vi "LFU Set File Pointer__ogtk.vi"(4 "error in (no error)":errorcluster, 5 "offset in (0)":dbl, 6 "pos mode (current)":enum16{"start", "end", "current"}(ring)=enum."current", 7 "handle":u32) -> (0 "error out":errorcluster, 1 "offset out":dbl, 3 "handle out":u32)   [LabVIEW 2018]
doc: "Low level utility function to change the current read/write pointer in a file using a double precision number to work for files larger than 2GB."
uses:
  kernel32.dll
panel:
  # "max offset is limited to about\n2^51 (1 000 000 000 000 000)  bytes\nto maintain full resolution of 1 bytes"
  # "LFU Set File Pointer.vi\n\nPlease visit http://www.OpenG.org to learn about the\nOpen Source LabVIEW software movement.\n\nNOTICE -- YOU MUST LEAVE THIS NOTICE IN PLACE.  PER THE TERMS OF THE LICENSE BELOW, YOU MAY SUBLICENSE THIS SOFTWARE \nIN ANY WAY THAT DOES NOT CONFLICT WITH THIS LICENSE.\n\n### BSD License (http://www.opensource.org/licenses/bsd-license.php) Begin ###\n\nCopyright (c) 2003, Rolf Kalbermatter <rolf.kalbermatter@citeng.com>\n\nAll rights reserved.\n\nRedistribution and use in source and binary forms, with or without modification, are permitted provided that the following conditions are met:\n\n    * Redistributions of source code must retain the above copyright notice, this list of conditions and the following disclaimer.\n    * Redistributions in binary form must reproduce the above copyright notice, this list of conditions and the following disclaimer in the \n       documentation and/or other materials provided with the distribution.\n    * Neither the name of SciWare, James Kring, Inc., nor the names of its contributors may be used to endorse or promote products derived \n       from this software without specific prior written permission.\n\nTHIS SOFTWARE IS PROVIDED BY THE COPYRIGHT HOLDERS AND CONTRIBUTORS \"AS IS\" AND ANY EXPRESS OR IMPLIED WARRANTIES, \nINCLUDING, BUT NOT LIMITED TO, THE IMPLIED WARRANTIES OF MERCHANTABILITY AND FITNESS FOR A PARTICULAR PURPOSE ARE \nDISCLAIMED. IN NO EVENT SHALL THE COPYRIGHT OWNER OR CONTRIBUTORS BE LIABLE FOR ANY DIRECT, INDIRECT, INCIDENTAL,\n SPECIAL, EXEMPLARY, OR CONSEQUENTIAL DAMAGES (INCLUDING, BUT NOT LIMITED TO, PROCUREMENT OF SUBSTITUTE GOODS OR \nSERVICES; LOSS OF USE, DATA, OR PROFITS; OR BUSINESS INTERRUPTION) HOWEVER CAUSED AND ON ANY THEORY OF LIABILITY, \nWHETHER IN CONTRACT, STRICT LIABILITY, OR TORT (INCLUDING NEGLIGENCE OR OTHERWISE) ARISING IN ANY WAY OUT OF THE USE \nOF THIS SOFTWARE, EVEN IF ADVISED OF THE POSSIBILITY OF SUCH DAMAGE.\n\n### BSD License End ###"
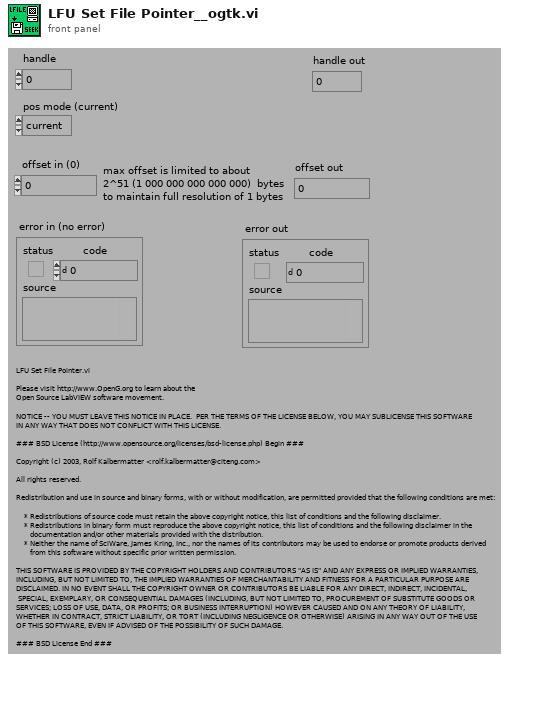
[diagram p1: front panel]
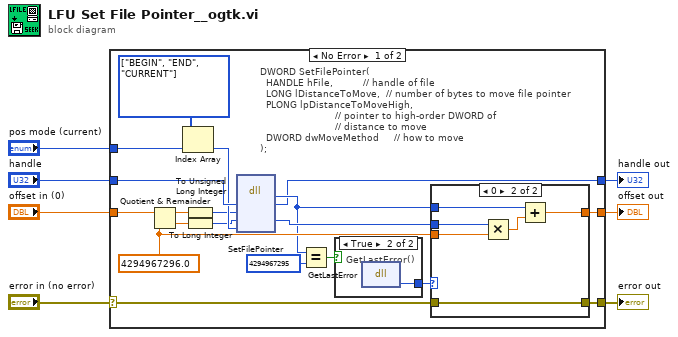
[diagram p0: block diagram]
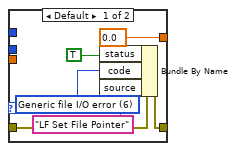
[diagram p2: hidden frame]
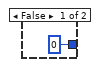
[diagram p3: hidden frame]
diagram:
  n1 = case shown="No Error" "error in (no error)" {
    selector: "error in (no error)" -> [w23 w41]
    tunnel: [w13 w43] -> w7
    tunnel: "handle" -> [w12 w43]
    tunnel: "pos mode (current)" -> [w26 _]
    tunnel: "offset in (0)" -> [w25 w42]
    tunnel: [w24 w42] -> w3
    tunnel: [w22 w41] -> w1
    frame No Error {
      w11 = enum16{"BEGIN", "CURRENT", "END"}[] [enum."BEGIN", enum."END", enum."CURRENT"] items=["BEGIN", "CURRENT", "END"]
      w18 = 4294967296.0
      # "DWORD SetFilePointer(\n  HANDLE hFile,          // handle of file\n  LONG lDistanceToMove,  // number of bytes to move file pointer\n  PLONG lpDistanceToMoveHigh,\n                         // pointer to high-order DWORD of \n                         // distance to move\n  DWORD dwMoveMethod     // how to move\n);"
      n2 = Quotient & Remainder(x=w25, y=w18) -> (x-y*floor(x/y)=w21:dbl, floor(x/y)=w20:dbl)
      n3 = Index Array(array=w11, index=w26) -> (element=w10:enum16{"BEGIN", "CURRENT", "END"})
      n4 = To Unsigned Long Integer(number=w21) -> (unsigned 32bit integer=w9:u32)
      n5 = To Long Integer(number=w20) -> (32bit integer=w8:i32)
      n6 = dll-call lib="kernel32.dll" fn="SetFilePointer"("handle"=w12, "dist"=w9, "lpDistHigh"=w8, "method"=w10) -> (w17:u32, "handle"=w13:u32, "lpDistHigh"=w19:i32)  [unwired: 5 in, 2 out]
      n7 = Equal?(x=w17, y=u32 4294967295) -> (x = y?=w16:bool)
      n8 = case shown="True" w16 {
        tunnel: [u32 0 w40] -> w14
        frame False {
        }
        frame True {
          # "GetLastError()"
          n9 = dll-call lib="kernel32.dll" fn="GetLastError"() -> (w40:u32)  [unwired: 3 in, 2 out]
        }
      }
      n10 = case shown="0" w14 {
        tunnel: w19 -> [_ w38]
        tunnel: w18 -> [_ w37]
        tunnel: [0.0 w35] -> w24
        tunnel: w17 -> [_ w34]
        tunnel: w23 -> [w27 w33]
        tunnel: [w31 w33] -> w22
        frame Default {
          w29 = 6 items=["No error", "Argument error", "Memory is full", "Out of zone", "End of file", "File already open", "Generic file I/O error", "File not found", "File permission error", "Disk is full", "Duplicate path", "Too many files open", "System feature not enabled", "Resource file not found", "Cannot add resource", "Resource not found", "Image not found", "Image memory error", "Pen does not exist", "Config type invalid", "Config token not found", "Config parse error", "Config memory error", "Bad external code format", "Bad external code offset", "External code not present", "Null window", "Destroy window error", "Null menu", "Print aborted", "Bad print record", "Print driver error", "Windows error during printing", "Memory error during printing", "Print dialog error", "Generic print error", "Invalid device refnum", "Device not found", "Device parameter error", "Device unit error", "Cannot open device", "Device call aborted", "Generic error", "Cancelled by user", "Object ID too low", "Object ID too high", "Object not in heap", "Unknown heap", "Unknown object (invalid DefProc)", "Unknown object (DefProc not in table)", "Message out of range", "Invalid (null) method", "Unknown message", "Manager call not supported", "Bad address", "Network operation in progress", "Network operation timed out", "Connection is busy", "Network attribute not supported", "Network error", "Address in use", "System out of memory", "Connection aborted", "Connection refused", "Not connected", "Already connected", "Connection closed", "Initialization error (interapplication manager)", "Bad occurrence", "Wait on unbound occurrence handler", "Occurrence queue overflow", "Datalog type conflict", "Unused", "Unrecognized type (interapplication manager)", "Memory corrupt", "Failed to make temporary DLL", "Old CIN version", "Drag socket not found", "Failed to load drop-object", "Failed to register OLE object", "Failed to release OLE object", "Format specifier type mismatch", "Unknown format specifier", "Too few format specifiers", "Too many format specifiers", "Scan failed", "Newer CIN version", "Error converting to variant", "Runtime menu error", "Password tampered", "Variant attribute not found", "Incompatible variant data type", "Event data is not available", "Event Store is not present", "Occurrence is not found", "Event Queue is not created", "Event info is not available", "Refnum passed is NULL", "Error retrieving Class GUID", "Error retrieving CoClass GUID", "Error retrieving TypeLib GUID.", "Bad built application magic bytes.", "Specific driver is different from the specific driver associated with the Logical Name.", "There is no session opened to the class driver.", "Max Error", "MAX - Error with config objects", "MAX - Error loading configuration", "MAX - Group not supported"]
          n11 = Bundle By Name(cluster=w27, "status"=TRUE, "code"=w29, "source"="LF Set File Pointer") -> (w31:errorcluster)
        }
        frame 0 {
          n12 = Multiply(x=w38, y=w37) -> (x*y=w36:dbl)
          n13 = Add(x=w34, y=w36) -> (x+y=w35:dbl)
        }
      }
    }
    frame Error {
    }
  }
  "handle out" <- w7
  "error out" <- w1
  "offset out" <- w3
